vi "Simulate Audio Hardware.vi"(6 "Command to Simulate":T2=enum."Mic Test - Simulate Read Microphone", 7 "error in (no error)":errorcluster, 9 "Simulation Data":T1={"PowerOn"=TRUE, "Battery"=TRUE, "Antenna"=TRUE, "Microphone"=TRUE, "Speakers"=TRUE, "Buttons"=TRUE, "LCD"=enum."Passing Image"}, 10 "Frequency":dbl=400000.0 format="%0.2f") -> (0 "error out":errorcluster, 3 "Response Signal Out":waveform(dbl))   [LabVIEW 2011]
uses:
  Audio Hardware Simulation Commands.ctl
  Simulation Data.ctl
  <vilib>/measure/macond.llb/FIR Filter for N Chan.vi
  <vilib>/measure/NI_MABase.lvlib
  <vilib>/measure/NI_MAPro.lvlib
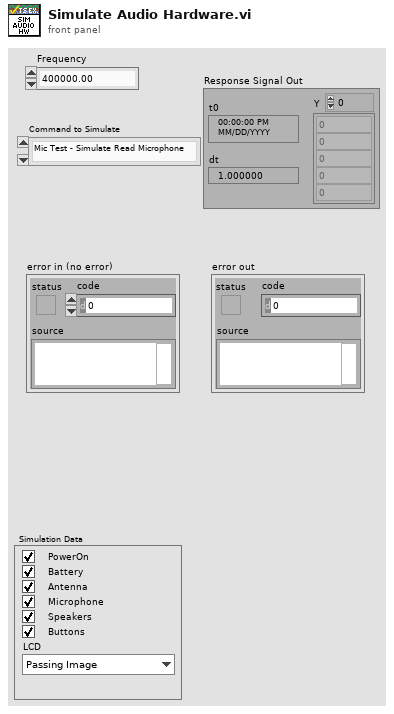
[diagram p1: front panel]
types:
  T1 = typedef "Simulation Data.ctl" = cluster{"PowerOn":bool, "Battery":bool, "Antenna":bool, "Microphone":bool, "Speakers":bool, "Buttons":bool, "LCD":enum16{"Passing Image", "Dead Pixels", "Incorrect Brightness"}}
  T2 = typedef "Audio Hardware Simulation Commands.ctl" = enum16{"Simulate Play Waveform", "Mic Test - Simulate Read Microphone", "Spkr Test - Simulate Read Microphone"}
  T3 = cluster{"PB Gain":dbl, "SB Gain":dbl, "Scale":bool, "Window":enum16{"None", "Hanning", "Hamming", "Triangular", "Blackman", "Exact Blackman", "Blackman-Harris", "Kaiser-Bessel", "Flat Top"}}
  T4 = cluster{"Topology":enum16{"Off", "FIR by Specification", "Equi-ripple FIR", "Windowed FIR"}, "Type":enum16{"Lowpass", "Highpass", "Bandpass", "Bandstop"}, "#Taps":i32, "Lower PB":dbl, "Upper PB":dbl, "Lower SB":dbl, "Upper SB":dbl}
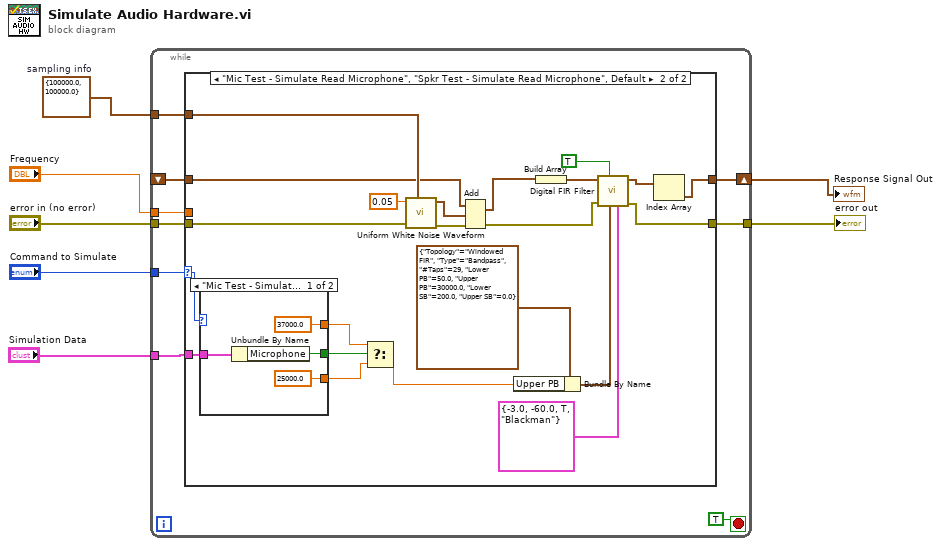
[diagram p0: block diagram]
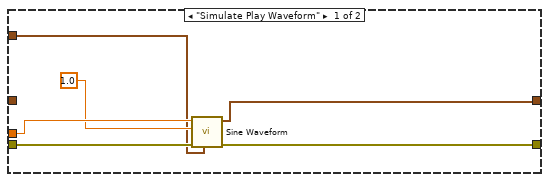
[diagram p2: hidden frame]
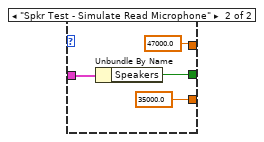
[diagram p3: hidden frame]
diagram:
  w1 = cluster{"Fs":dbl, "#s":dbl} {"Fs"=100000.0, "#s"=100000.0}  # sampling info
  n1 = while {
    tunnel: [w16] -> w7
    tunnel: "error in (no error)" -> [w15]
    tunnel: "Command to Simulate" -> [w14]
    tunnel: "Frequency" -> [w12]
    shift-right: [w11] -> w2
    shift-left: _ -> [w10]
    tunnel: "Simulation Data" -> [w9]
    tunnel: w1 -> [w8]
    stop <- TRUE stop-if-true
    n2 = case shown="\"Mic Test - Simulate Read Microphone\", \"Spkr Test - Simulate Read Microphone\", Default" w14 {
      selector: w14 -> [_ w40]
      tunnel: [w19 w42] -> w16
      tunnel: w15 -> [w20 w38]
      tunnel: w12 -> [w22 _]
      tunnel: [w18 w31] -> w11
      tunnel: w10 -> [_ w29]
      tunnel: w9 -> [_ w41]
      tunnel: w8 -> [w17 w37]
      frame "Simulate Play Waveform" {
        n3 = call <vilib>:"Sine Waveform.vi"("sampling info"=w17, "error in (no error)"=w20, "amplitude"=1.0, "frequency"=w22) -> ("error out"=w19:errorcluster, "signal out"=w18:waveform(dbl))  [unwired: 6 in]
      }
      frame "Mic Test - Simulate Read Microphone", "Spkr Test - Simulate Read Microphone", Default {
        n4 = case shown="\"Mic Test - Simulate Read Microphone\", Default" w40 {
          tunnel: w41 -> [w48 w52]
          tunnel: [w47 w51] -> w39
          tunnel: [25000.0 ("f") 35000.0 ("f")] -> w24
          tunnel: [37000.0 ("amplitude") 47000.0 ("amplitude")] -> w23
          frame "Mic Test - Simulate Read Microphone", Default {
            n5 = Unbundle By Name(w48) -> ("Microphone"=w47:bool)
          }
          frame "Spkr Test - Simulate Read Microphone" {
            n6 = Unbundle By Name(w52) -> ("Speakers"=w51:bool)
          }
        }
        n7 = Select(t=w23, s=w39, f=w24) -> (s? t:f=w28:dbl)
        n8 = call <vilib>:"Uniform White Noise Waveform.vi"("sampling info"=w37, "error in (no error)"=w38, "amplitude"=0.05) -> ("error out"=w36:errorcluster, "signal out"=w32:waveform(dbl))  [unwired: 7 in]
        n9 = Add(1:w32, 2:w29, 4:w36) -> (0:w30:waveform(dbl), 3:w35:errorcluster)
        n10 = Bundle By Name(cluster=T4 {"Topology"=enum."Windowed FIR", "Type"=enum."Bandpass", "#Taps"=29, "Lower PB"=50.0, "Upper PB"=30000.0, "Lower SB"=200.0, "Upper SB"=0.0} ("FIR filter specifications"), "Upper PB"=w28) -> (w26:T4)
        n11 = Build Array(w30) -> (w34:waveform(dbl)[])
        n12 = call-poly <vilib>:"Digital FIR Filter.vi"("optional FIR filter specifications"=T3 {"PB Gain"=-3.0, "SB Gain"=-60.0, "Scale"=TRUE, "Window"=enum."Blackman"}, "FIR filter specifications"=w26, "reset filters"=TRUE, "error in (no error)"=w35, "signal(s) in"=w34) -> ("error out"=w42:errorcluster, "signal(s) out"=w33:waveform(dbl)[])  [unwired: 4 in, 1 out]
        n13 = Index Array(array=w33) -> (element=w31:waveform(dbl))  [unwired: 1 in]
      }
    }
  }
  "error out" <- w7
  "Response Signal Out" <- w2
